vi "ListRecursiveWithPriorityWithPattern.vi"(0 "basePath":path=path "D:/data/Prosis/Schnell", 1 "pattern":string, 2 "Wait":i32=100, 13 "ignore Files in Directorys with subdirectorys":bool) -> (4 "fileArray":path[](array[path]), 6 "dirArray":path[](array[path]))   [LabVIEW 2013]
panel:
  in  "stop":bool
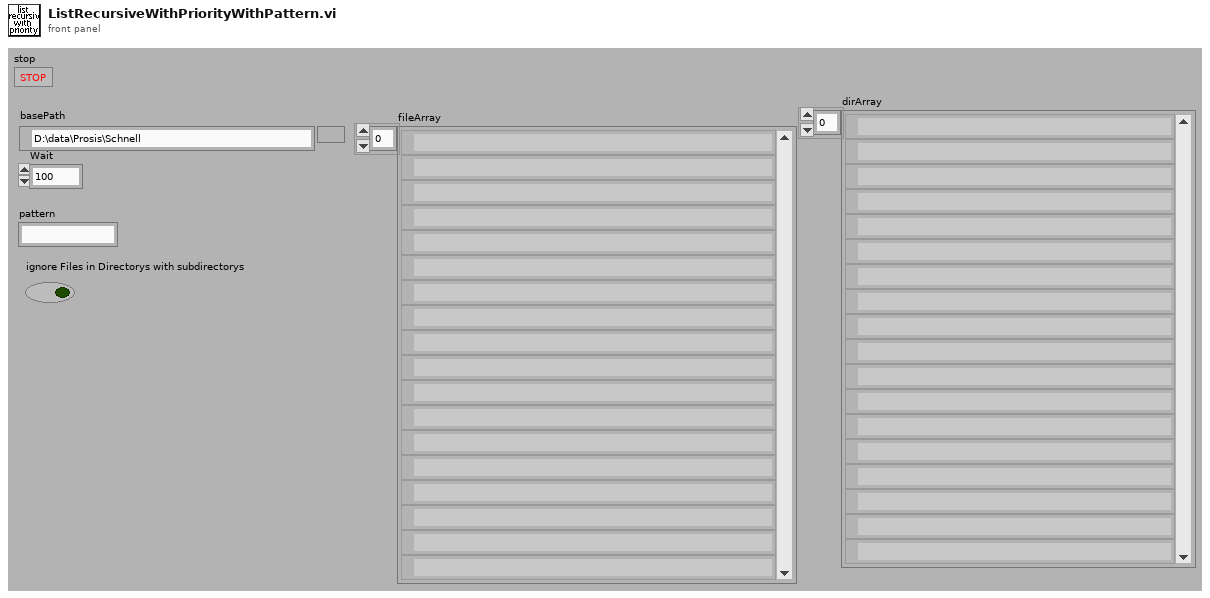
[diagram p1: front panel]
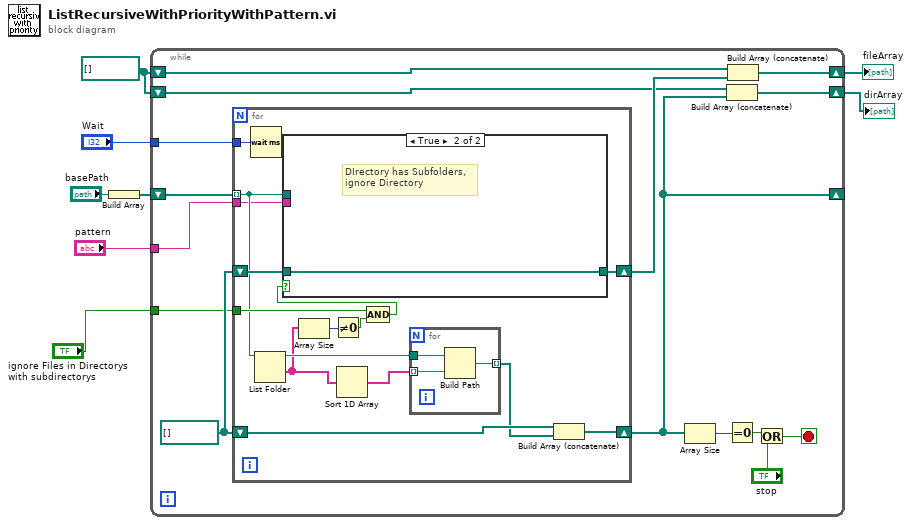
[diagram p0: block diagram]
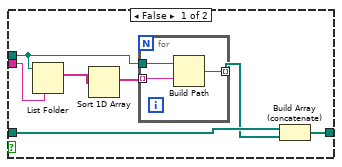
[diagram p2: hidden frame]
diagram:
  w5 = path[] [] ("Array")
  n1 = Build Array("basePath") -> (w7:path[])
  n2 = while {
    shift-right: [w17] -> w4
    shift-left: w5 -> [w18]
    shift-right: [w11] -> _
    shift-left: w7 -> [w23]
    tunnel: "Wait" -> [w14]
    shift-right: [w12] -> w3
    shift-left: w5 -> [w13]
    tunnel: "pattern" -> [w10]
    tunnel: "ignore Files in Directorys with subdirectorys" -> [w9]
    stop <- w21 stop-if-true
    w16 = path[] []
    n3 = for {
      tunnel: w23 -> [w25] mode=indexing
      shift-right: [w38] -> w11
      shift-left: w16 -> [w37]
      shift-right: [w35] -> w15
      shift-left: w16 -> [w34]
      tunnel: w14 -> [w33]
      tunnel: w10 -> [w24]
      tunnel: w9 -> [w27]
      n4 = Wait (ms)(milliseconds to wait=w33) -> ()  [unwired: 1 out]
      n5 = List Folder(path=w25) -> (path out=w32:path, folder names=w30:string[])  [unwired: 3 in, 2 out]
      n6 = Array Size(array=w30) -> (size(s)=w29:i32)
      n7 = Not Equal To 0?(x=w29) -> (x != 0?=w28:bool)
      n8 = Sort 1D Array(array=w30) -> (sorted array=w31:string[])
      n9 = Compound Arithmetic op=AND(w27, w28) -> (w26:bool)
      n10 = case shown="True" w26 {
        tunnel: [w45 w49] -> w35
        tunnel: w34 -> [w44 w49]
        tunnel: w25 -> [w40 _]
        tunnel: w24 -> [w41 _]
        frame False {
          n11 = List Folder(path=w40, pattern=w41) -> (filenames=w39:string[])  [unwired: 2 in, 3 out]
          n12 = Sort 1D Array(array=w39) -> (sorted array=w42:string[])
          n13 = for {
            tunnel: w40 -> [w48]
            tunnel: w42 -> [w47] mode=indexing
            tunnel: [w46] -> w43 mode=indexing
            n14 = Build Path(base path=w48, name or relative path=w47) -> (appended path=w46:path)
          }
          n15 = Build Array (concatenate)(w44, w43) -> (w45:path[])
        }
        frame True {
          # "DIrectory has Subfolders,\nignore Directory"
        }
      }
      n16 = for {
        tunnel: w32 -> [w52]
        tunnel: w31 -> [w51] mode=indexing
        tunnel: [w50] -> w36 mode=indexing
        n17 = Build Path(base path=w52, name or relative path=w51) -> (appended path=w50:path)
      }
      n18 = Build Array (concatenate)(w37, w36) -> (w38:path[])
    }
    n19 = Array Size(array=w11) -> (size(s)=w22:i32)
    n20 = Build Array (concatenate)(w13, w11) -> (w12:path[])
    n21 = Equal To 0?(x=w22) -> (x = 0?=w19:bool)
    n22 = Build Array (concatenate)(w18, w15) -> (w17:path[])
    n23 = Or(x=w19, y="stop") -> (x .or. y?=w21:bool)
  }
  "fileArray" <- w4
  "dirArray" <- w3
